vi "Safety_FGV.vi"(8 "Error In":errorcluster, 11 "Action":T2) -> (0 "Error Out":errorcluster, 2 "LED":T1, 3 "Safetymsg":string)   [LabVIEW 2021, in "Signal.lvlib"]
doc: "This FGV is used to check if the voltage is safe (under 50V), if it is not the FGV is used to make blinking effect."
uses:
  Signal.lvlib
  Tipski Definicii/danger.ctl
  Tipski Definicii/Signal Values.ctl
  Tipski Definicii/Unit.ctl
panel:
  # "Output"
  # "Input"
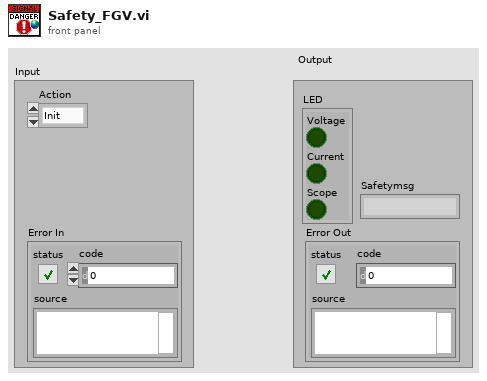
[diagram p1: front panel]
types:
  T1 = cluster{"Voltage":bool, "Current":bool, "Scope":bool}
  T2 = typedef "danger.ctl" = enum16{"Init", "Check"}
  T3 = typedef "Unit.ctl" = enum16{"Init", "Add", "Read"}
  T4 = typedef "Signal Values.ctl" = enum16{"Init", "Add V/A string", "Add Hz string", "Get Strings and Values", "Reset", "Add Offset", "Add Waveform", "Add Phase"}
  T5 = cluster{"Amp String":string, "Amp Value":dbl, "Hz Value Out":dbl, "Waveform Out":enum16{"Sine Wave", "Triangle Wave", "Square Wave", "Sawtooth Wave"}, "Offset Out":dbl, "Phase Out":dbl, "Signal String":string, "Signal":waveform(dbl)}
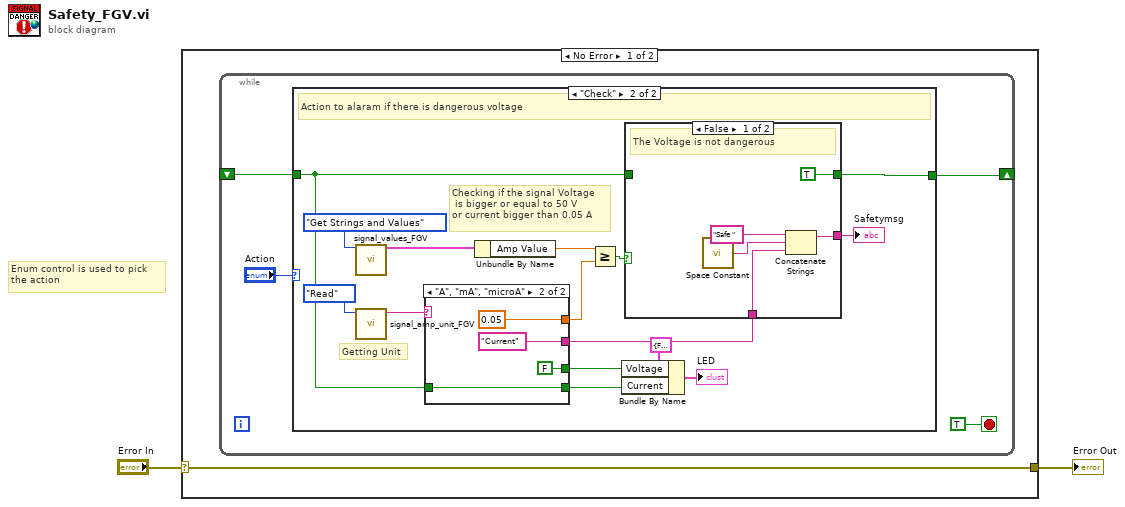
[diagram p0: block diagram]
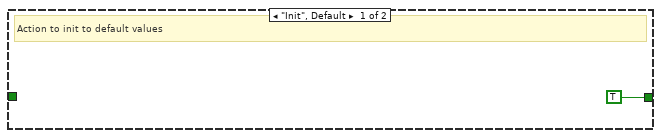
[diagram p2: hidden frame]
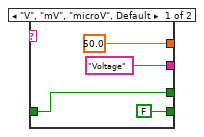
[diagram p3: hidden frame]
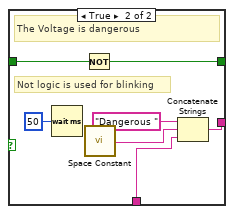
[diagram p4: hidden frame]
diagram:
  # "Enum control is used to pick \nthe action"
  n1 = case shown="No Error" "Error In" {
    selector: "Error In" -> [w3 w44]
    tunnel: [w3 w44] -> w1
    frame No Error {
      n2 = while {
        shift-right: [w5] -> _
        shift-left: _ -> [w4]
        stop <- TRUE stop-if-true
        n3 = case shown="\"Check\"" "Action" {
          tunnel: [TRUE w22] -> w5
          tunnel: w4 -> [_ w12]
          frame "Init", Default {
            # "Action to init to default values"
          }
          frame "Check" {
            # "Getting Unit"
            # "Checking if the signal Voltage\n is bigger or equal to 50 V\nor current bigger than 0.05 A"
            # "Action to alaram if there is dangerous voltage"
            n4 = call "signal_values_FGV.vi"("Action"=Signal_Values."Get Strings and Values") -> ("Signal"=w20:T5)  [unwired: 13 in, 1 out]
            n5 = call "signal_amp_unit_FGV.vi"("Action"=Unit."Read") -> ("Unit (Not F)"=w16:string)  [unwired: 8 in, 2 out]
            n6 = case shown="\"A\", \"mA\", \"microA\"" w16 {
              tunnel: [50.0 0.05] -> w15
              tunnel: ["Voltage" "Current"] -> w14
              tunnel: w12 -> [w24 w28]
              tunnel: [w24 FALSE] -> w11
              tunnel: [FALSE ("Current") w28] -> w10
              frame "V", "mV", "microV", Default {
              }
              frame "A", "mA", "microA" {
              }
            }
            n7 = Unbundle By Name(w20) -> ("Amp Value"=w19:dbl)
            n8 = Greater Or Equal?(x=w19, y=w15) -> (x >= y?=w23:bool)
            n9 = Bundle By Name(cluster=T1 {"Voltage"=FALSE, "Current"=FALSE, "Scope"=FALSE}, "Voltage"=w11, "Current"=w10) -> (→"LED":T1)
            n10 = case shown="False" w23 {
              tunnel: [TRUE w42] -> w22
              tunnel: w12 -> [_ w43]
              tunnel: [w34 w39] -> w21
              tunnel: w14 -> [w32 w37]
              frame False {
                # "The Voltage is not dangerous"
                n11 = call <vilib>:"Space Constant.vi"() -> ("String"=w33:string)
                n12 = Concatenate Strings("Safe ", w33, w32) -> (w34:string)
              }
              frame True {
                # "Not logic is used for blinking"
                # "The Voltage is dangerous"
                n13 = Wait (ms)(milliseconds to wait=u32 50) -> ()  [unwired: 1 out]
                n14 = Not(x=w43) -> (.not. x?=w42:bool)
                n15 = call <vilib>:"Space Constant.vi"() -> ("String"=w38:string)
                n16 = Concatenate Strings("Dangerous ", w38, w37) -> (w39:string)
              }
            }
            "Safetymsg" <- w21
          }
        }
      }
    }
    frame Error {
    }
  }
  "Error Out" <- w1
